vi "Log In Dialog.vi"(8 "error in (no error)":errorcluster) -> (0 "error out":errorcluster, 2 "Result":T1={"username"="admin", "password"="", "save credentials to disk"=FALSE}, 3 "Cancelled?":bool)   [LabVIEW 2017]
doc: "Use this template to create a dialog box with event handling."
panel:
  in  "save credentials to disk":bool
  in  "password":string
  in  "username":string
  in  "Cancel":bool
  in  "OK":bool=TRUE
  # "Username"
  # "Password"
  # "Save Credentials to Disk"
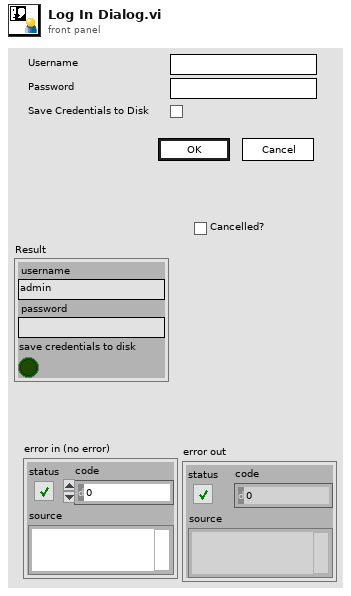
[diagram p1: front panel]
types:
  T1 = cluster{"username":string, "password":string, "save credentials to disk":bool}
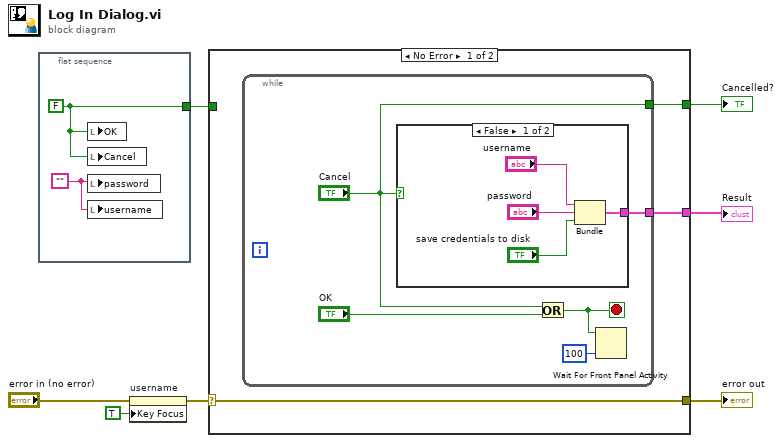
[diagram p0: block diagram]
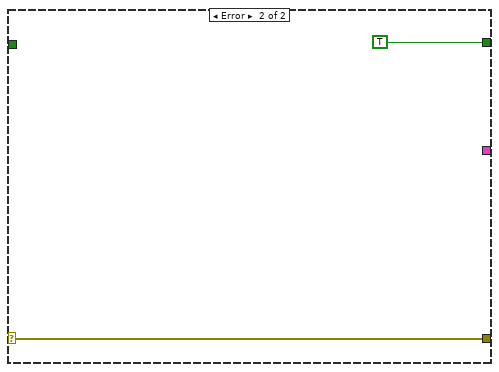
[diagram p3: hidden frame]
diagram:
  n1 = flat-sequence {
    tunnel: [w9] -> w4
    frame #0 {
      w8 = ""
      w9 = FALSE
      n2 = local write "OK"(w9) -> ()
      n3 = local write "Cancel"(w9) -> ()
      n4 = local write "password"(w8) -> ()
      n5 = local write "username"(w8) -> ()
    }
  }
  n6 = property on="username" class="Str"(error in="error in (no error)", "Key Focus"=TRUE) -> (error out=w2:errorcluster)  [unwired: 1 in, 1 out]
  n7 = case shown="No Error" w2 {
    selector: w2 -> [w10 w23]
    tunnel: [w12 TRUE ("Cancel")] -> w7
    tunnel: [w11 _] -> w6
    tunnel: [w10 w23] -> w5
    tunnel: w4 -> [_ _]
    frame No Error {
      n8 = while {
        tunnel: ["Cancel"] -> w12
        tunnel: [w15] -> w11
        stop <- w13 stop-if-true
        n9 = case shown="False" "Cancel" {
          tunnel: [w18 _] -> w15
          frame False {
            n10 = Bundle("username"="username", "password"="password", "save credentials to disk"="save credentials to disk") -> (w18:T1)  [unwired: 1 in]
          }
          frame True {
          }
        }
        n11 = Or(x="Cancel", y="OK") -> (x .or. y?=w13:bool)
        n12 = Wait For Front Panel Activity(1:100 ("timeout ms (-1 never timeout)"), 3:w13) -> ()  [unwired: 1 in, 1 out]
      }
    }
    frame Error {
    }
  }
  "Cancelled?" <- w7
  "Result" <- w6
  "error out" <- w5
